vi "2_CONFIGURE_OUTPUT_.vi"() -> ()   [LabVIEW 2020]
panel:
  out "resulting string":string
  in  "Auto Output-Off (F: Disable)":bool
  in  "Channel (0: Channel 1)":i32(ring) items=["Channel 1", "Channel 2"]
  in  "Enable High Capacitance (F: Disable)":bool
  in  "Low Terminal State (1: Ground)":i32(ring)=1 items=["Float", "Ground"]
  in  "Auto Output-On (T: Enable)":bool=TRUE
  in  "Output-Off Status (2: Normal)":i32(ring)=2 items=["Zero", "HIZ", "Normal"]
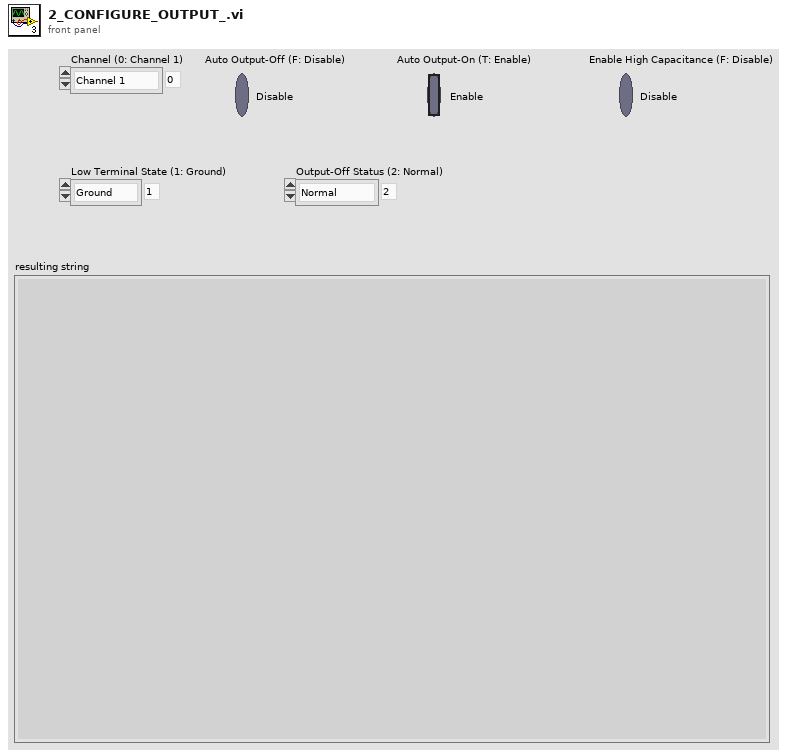
[diagram p1: front panel]
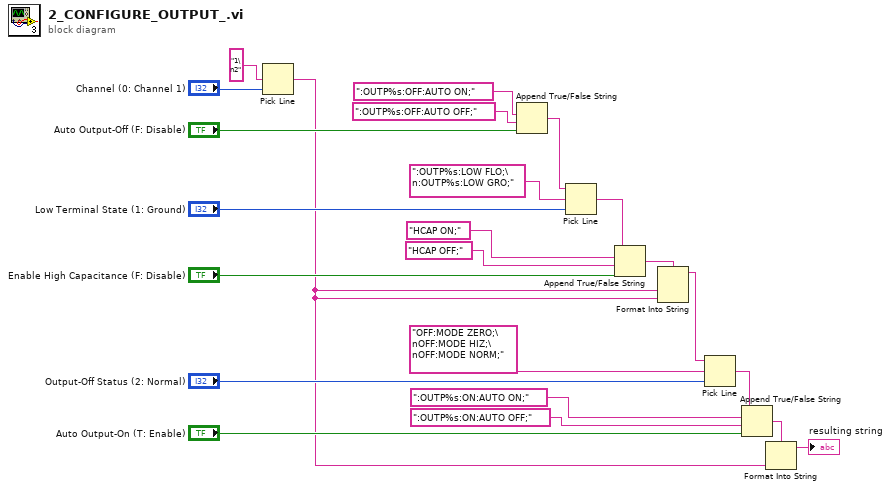
[diagram p0: block diagram]
diagram:
  n1 = Pick Line(multi-line string="1\n2" ("string (\"\")"), line index="Channel (0: Channel 1)") -> (output string=w2:string)  [unwired: 1 in]
  n2 = Append True/False String(1:"Auto Output-Off (F: Disable)", 2:":OUTP%s:OFF:AUTO OFF;", 3:":OUTP%s:OFF:AUTO ON;") -> (0:w4:string)  [unwired: 1 in]
  n3 = Pick Line(string ("")=w4, multi-line string=":OUTP%s:LOW FLO;\n:OUTP%s:LOW GRO;", line index="Low Terminal State (1: Ground)") -> (output string=w15:string)
  n4 = Append True/False String(1:"Enable High Capacitance (F: Disable)", 2:"HCAP OFF;", 3:"HCAP ON;", 4:w15) -> (0:w3:string)
  n5 = Format Into String(format string=w3, w2, w2) -> (resulting string=w11:string)  [unwired: 2 in, 1 out]
  n6 = Pick Line(string ("")=w11, multi-line string="OFF:MODE ZERO;\nOFF:MODE HIZ;\nOFF:MODE NORM;", line index="Output-Off Status (2: Normal)") -> (output string=w21:string)
  n7 = Append True/False String(1:"Auto Output-On (T: Enable)", 2:":OUTP%s:ON:AUTO OFF;", 3:":OUTP%s:ON:AUTO ON;", 4:w21) -> (0:w10:string)
  n8 = Format Into String(format string=w10, w2) -> (resulting string=→"resulting string":string)  [unwired: 2 in, 1 out]
